vi "OC_ADC_core.vi"(10 "value":u8 format="%02x", 11 "registers":T1={"A"=0, "X"=0, "Y"=0, "SP"=253, "PC"=0, "P"=36} {"P" format="%08b"; "PC" format="%04x"; "SP" format="%02x"; "Y" format="%02x"; "X" format="%02x"; "A" format="%02x"}) -> (3 "registers":T1={"A"=0, "X"=0, "Y"=0, "SP"=253, "PC"=0, "P"=36} {"P" format="%08b"; "PC" format="%04x"; "SP" format="%02x"; "Y" format="%02x"; "X" format="%02x"; "A" format="%02x"})   [LabVIEW 2018]
uses:
  CPU_registers.ctl
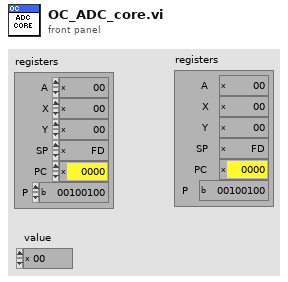
[diagram p1: front panel]
types:
  T1 = typedef "CPU_registers.ctl" = cluster{"A":u8, "X":u8, "Y":u8, "SP":u8, "PC":u16, "P":u8}
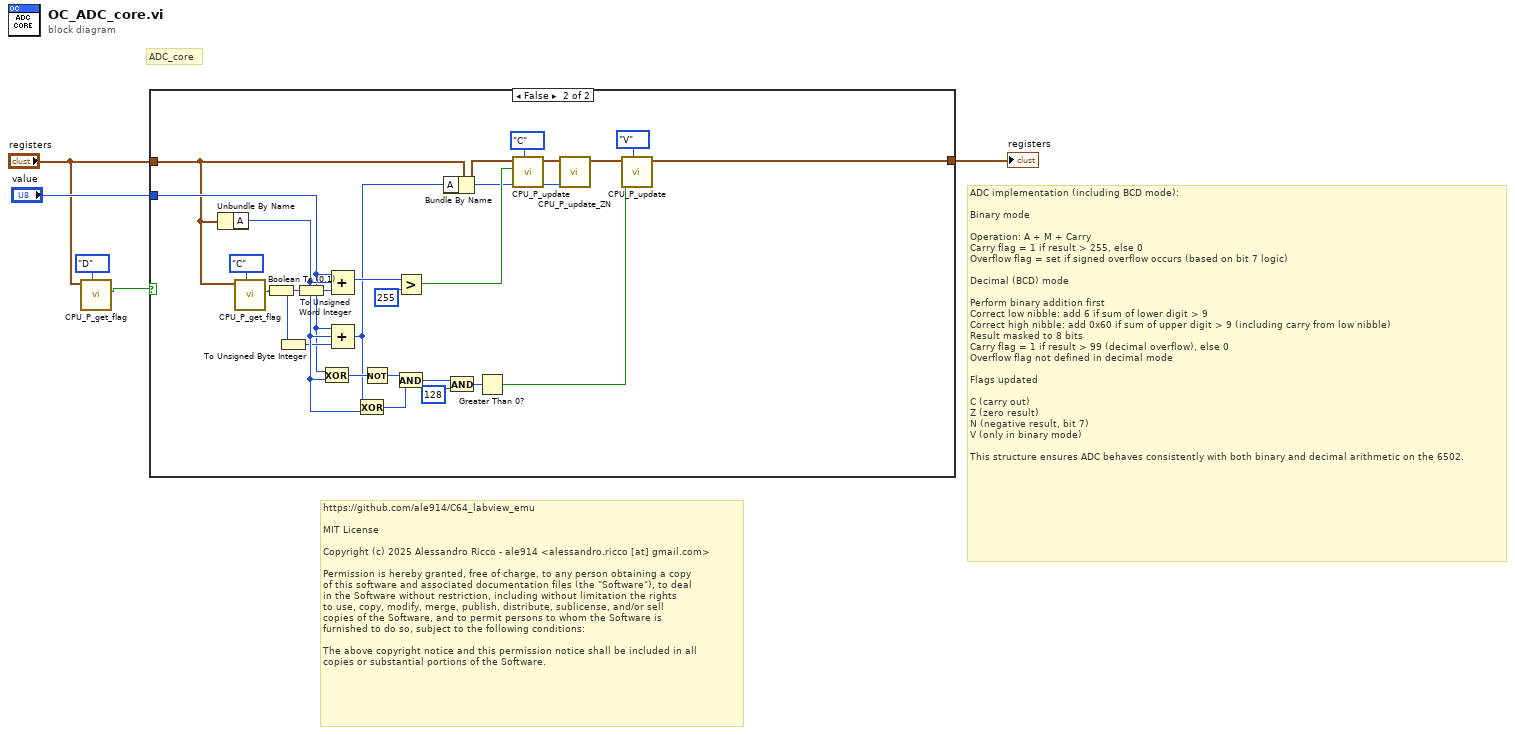
[diagram p0: block diagram]
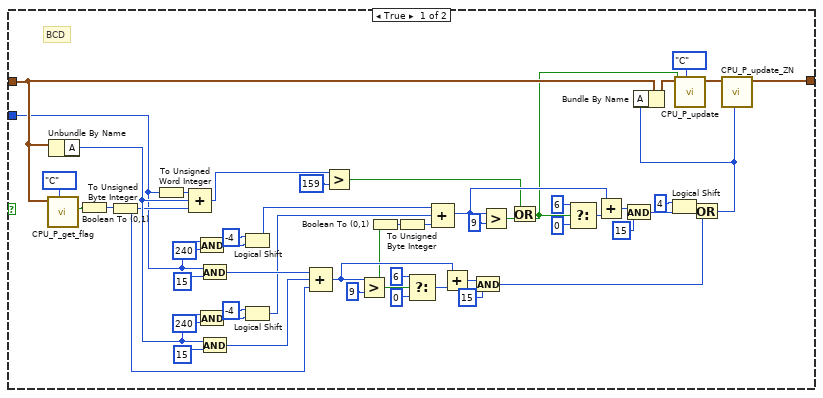
[diagram p2: hidden frame]
diagram:
  # "ADC implementation (including BCD mode):\n\nBinary mode\n\nOperation: A + M + Carry\nCarry flag = 1 if result > 255, else 0\nOverflow flag = set if signed overflow occurs (based on bit 7 logic)\n\nDecimal (BCD) mode\n\nPerform binary addition first\nCorrect low nibble: add 6 if sum of lower digit > 9\nCorrect high nibble: add 0x60 if sum of upper digit > 9 (including carry from low nibble)\nResult masked to 8 bits\nCarry flag = 1 if result > 99 (decimal overflow), else 0\nOverflow flag not defined in decimal mode\n\nFlags updated\n\nC (carry out)\nZ (zero result)\nN (negative result, bit 7)\nV (only in binary mode)\n\nThis structure ensures ADC behaves consistently with both binary and decimal arithmetic on the 6502."
  # "https://github.com/ale914/C64_labview_emu\n\nMIT License\n\nCopyright (c) 2025 Alessandro Ricco - ale914 <alessandro.ricco [at] gmail.com>\n\nPermission is hereby granted, free of charge, to any person obtaining a copy\nof this software and associated documentation files (the \"Software\"), to deal\nin the Software without restriction, including without limitation the rights\nto use, copy, modify, merge, publish, distribute, sublicense, and/or sell\ncopies of the Software, and to permit persons to whom the Software is\nfurnished to do so, subject to the following conditions:\n\nThe above copyright notice and this permission notice shall be included in all\ncopies or substantial portions of the Software."
  # "ADC_core"
  n1 = call "CPU_P_get_flag.vi"("flag"=enum8{"C", "Z", "I", "D", "B", "V", "N"}."D", "registers"="registers") -> ("Value"=w1:bool)  [unwired: 8 in, 1 out]
  n2 = case shown="False" w1 {
    tunnel: [w50 w59] -> w5
    tunnel: "value" -> [w7 w58]
    tunnel: "registers" -> [w49 w57]
    frame True {
      # "BCD"
      n3 = call "CPU_P_get_flag.vi"("flag"=enum8{"C", "Z", "I", "D", "B", "V", "N"}."C", "registers"=w49) -> ("Value"=w55:bool)  [unwired: 8 in, 1 out]
      n4 = Unbundle By Name(w49) -> ("A"=w40:u8)
      n5 = Boolean To (0,1)(Boolean=w55) -> (0, 1=w54:i16)
      n6 = To Unsigned Byte Integer(number=w54) -> (unsigned 8bit integer=w37:u8)
      n7 = To Unsigned Word Integer(number=w7) -> (unsigned 16bit integer=w8:u16)
      n8 = Compound Arithmetic op=ADD(w8, w40, w37) -> (w9:u16)
      n9 = And(x=w7, y=u8 240) -> (x .and. y?=w46:u8)
      n10 = And(x=w40, y=u8 240) -> (x .and. y?=w43:u8)
      n11 = And(x=w7, y=u8 15) -> (x .and. y?=w39:u8)
      n12 = And(x=w40, y=u8 15) -> (x .and. y?=w38:u8)
      n13 = Logical Shift(y=i16 -4, x=w46) -> (x << y=w31:u8)
      n14 = Logical Shift(y=i16 -4, x=w43) -> (x << y=w30:u8)
      n15 = Compound Arithmetic op=ADD(w39, w38, w37) -> (w32:u8)
      n16 = Greater?(x=w9, y=u16 159) -> (0:w6:bool)
      n17 = Greater?(x=w32, y=u8 9) -> (0:w29:bool)
      n18 = Boolean To (0,1)(Boolean=w29) -> (0, 1=w28:i16)
      n19 = To Unsigned Byte Integer(number=w28) -> (unsigned 8bit integer=w27:u8)
      n20 = Select(t=u8 6 ("y"), s=w29, f=u8 0 ("y")) -> (s? t:f=w33:u8)
      n21 = Compound Arithmetic op=ADD(w31, w30, w27) -> (w22:u8)
      n22 = Add(x=w32, y=w33) -> (x+y=w20:u8)
      n23 = And(x=w20, y=u8 15) -> (x .and. y?=w14:u8)
      n24 = Greater?(x=w22, y=u8 9) -> (0:w13:bool)
      n25 = Or(x=w6, y=w13) -> (x .or. y?=w11:bool)
      n26 = Select(t=u8 6 ("y"), s=w11, f=u8 0 ("y")) -> (s? t:f=w26:u8)
      n27 = Add(x=w22, y=w26) -> (x+y=w18:u8)
      n28 = And(x=w18, y=u8 15) -> (x .and. y?=w16:u8)
      n29 = Logical Shift(y=i16 4, x=w16) -> (x << y=w15:u8)
      n30 = Or(x=w15, y=w14) -> (x .or. y?=w12:u8)
      n31 = Bundle By Name(cluster=w49, "A"=w12) -> (w53:T1)
      n32 = call "CPU_P_update.vi"("flag"=enum8{"C", "Z", "I", "D", "B", "V", "N"}."C", "Value"=w11, "registers"=w53) -> ("registers"=w52:T1)  [unwired: 8 in]
      n33 = call "CPU_P_update_ZN.vi"("value"=w12, "registers"=w52) -> ("registers"=w50:T1)  [unwired: 9 in]
    }
    frame False {
      n34 = Unbundle By Name(w57) -> ("A"=w69:u8)
      n35 = call "CPU_P_get_flag.vi"("flag"=enum8{"C", "Z", "I", "D", "B", "V", "N"}."C", "registers"=w57) -> ("Value"=w80:bool)  [unwired: 8 in, 1 out]
      n36 = Boolean To (0,1)(Boolean=w80) -> (0, 1=w68:i16)
      n37 = To Unsigned Byte Integer(number=w68) -> (unsigned 8bit integer=w67:u8)
      n38 = To Unsigned Word Integer(number=w68) -> (unsigned 16bit integer=w79:u16)
      n39 = Exclusive Or(1:w69, 2:w58) -> (0:w70:u8)
      n40 = Compound Arithmetic op=ADD(w58, w69, w79) -> (w75:u16)
      n41 = Compound Arithmetic op=ADD(w58, w69, w67) -> (w60:u8)
      n42 = Exclusive Or(1:w69, 2:w60) -> (0:w65:u8)
      n43 = Not(x=w70) -> (.not. x?=w66:u8)
      n44 = Greater?(x=w75, y=u16 255) -> (0:w73:bool)
      n45 = And(x=w66, y=w65) -> (x .and. y?=w64:u8)
      n46 = Bundle By Name(cluster=w57, "A"=w60) -> (w78:T1)
      n47 = And(x=w64, y=u8 128) -> (x .and. y?=w62:u8)
      n48 = Greater Than 0?(x=w62) -> (x > 0?=w61:bool)
      n49 = call "CPU_P_update.vi"("flag"=enum8{"C", "Z", "I", "D", "B", "V", "N"}."C", "Value"=w73, "registers"=w78) -> ("registers"=w77:T1)  [unwired: 8 in]
      n50 = call "CPU_P_update_ZN.vi"("value"=w60, "registers"=w77) -> ("registers"=w71:T1)  [unwired: 9 in]
      n51 = call "CPU_P_update.vi"("flag"=enum8{"C", "Z", "I", "D", "B", "V", "N"}."V", "Value"=w61, "registers"=w71) -> ("registers"=w59:T1)  [unwired: 8 in]
    }
  }
  "registers" <- w5
